vi "PID Coerce Into Range.vi"(8 "Deadband":dbl, 9 "Error":dbl, 11 "Output":dbl) -> (0 "Tolerable?":bool, 3 "upper limit":dbl)   [LabVIEW 2014]
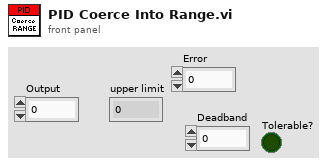
[diagram p1: front panel]
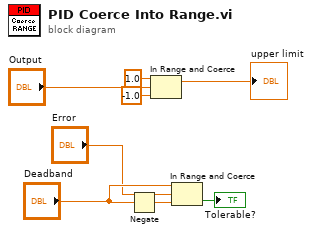
[diagram p0: block diagram]
diagram:
  n1 = Negate(x="Deadband") -> (-x=w4:dbl)
  n2 = In Range and Coerce(upper limit=1.0, x="Output", lower limit=-1.0) -> (coerced(x)=→"upper limit":dbl)  [unwired: 1 out]
  n3 = In Range and Coerce(upper limit="Deadband", x="Error", lower limit=w4) -> (In Range?=→"Tolerable?":bool)  [unwired: 1 out]
